vi "Close.vi"(8 "error in (no error)":errorcluster, 11 "LibreVNA in":refnum<class "LibreVNA.lvclass">) -> (0 "error out":errorcluster, 3 "LibreVNA out":refnum<class "LibreVNA.lvclass">)   [LabVIEW 2023, in "LibreVNA.lvclass"]
uses:
  LibreVNA.lvclass
  LibreVNA.lvclass/LibreVNA.ctl
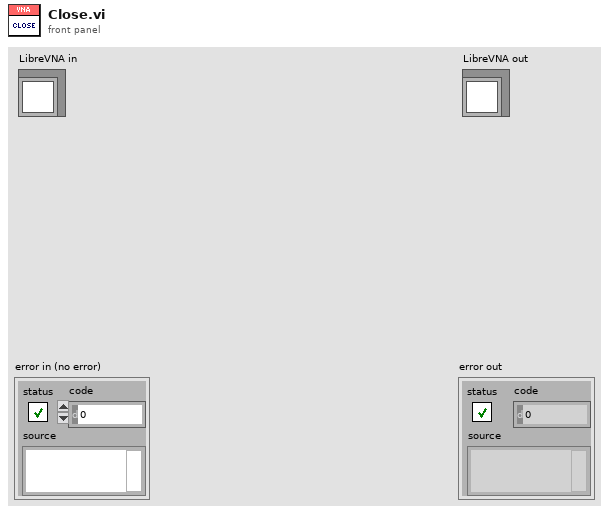
[diagram p1: front panel]
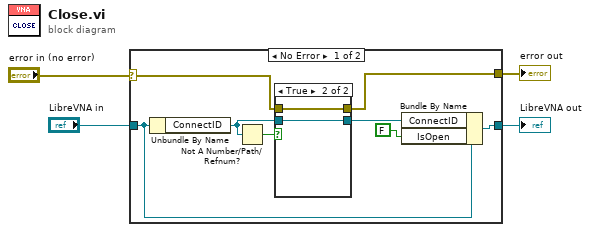
[diagram p0: block diagram]
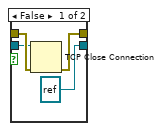
[diagram p2: hidden frame]
diagram:
  n1 = case shown="No Error" "error in (no error)" {
    selector: "error in (no error)" -> [w11 w20]
    tunnel: [w10 w20] -> w3
    tunnel: [w9 w19] -> w1
    tunnel: "LibreVNA in" -> [w12 w19]
    frame No Error {
      n2 = Unbundle By Name(w12) -> ("ConnectID"=w8:refnum<k5>)
      n3 = Not A Number/Path/Refnum?(number/path/refnum=w8) -> (NaN/Path/Refnum?=w7:bool)
      n4 = case shown="True" w7 {
        tunnel: w11 -> [w16 w17]
        tunnel: [w15 w17] -> w10
        tunnel: w8 -> [w14 w18]
        tunnel: [refnum<k5> refnum ("ConnectID") w18] -> w6
        frame False {
          n5 = TCP Close Connection(connection ID=w14, error in (no error)=w16) -> (error out=w15:errorcluster)  [unwired: 1 in, 1 out]
        }
        frame True {
        }
      }
      n6 = Bundle By Name(cluster=w12, "ConnectID"=w6, "IsOpen"=FALSE) -> (w9:refnum<class "LibreVNA.lvclass">)
    }
    frame Error {
    }
  }
  "error out" <- w3
  "LibreVNA out" <- w1
